vi "TEST_bench_X_minus_Nx_times_ye_singleAxis.vi"(6 "NS + 1":u8=9, 8 "xk_1_2_mem":fxp<+/-,32,5>[](array[numeric])=[0.0, 0.0, 0.0, 0.0, 0.0, 0.0, 0.0, 0.0, 0.0, 0.0, 0.0, 0.0, 0.0, 0.0, 0.0, 0.0, 0.0, 0.0, 0.0, 0.0, 0.0, 0.0, 0.0, 0.0, 0.0, 0.0, 0.0, 0.0, 0.0, 0.0, 0.0, 0.0, 0.0, 0.0, 0.0, 0.0, 0.0, 0.0, 0.0, 0.0, 0.0, 0.0, 0.0, 0.0, 0.0, 0.0, 0.0, 0.0, 0.0, 0.0], 11 "Nx":fxp<+/-,32,5>[](array[numeric])=[0.0, 0.0, 0.0, 0.0, 0.0, 0.0, 0.0, 0.0, 0.0, 0.0, 0.0, 0.0, 0.0, 0.0, 0.0, 0.0, 0.0, 0.0, 0.0, 0.0, 0.0, 0.0, 0.0, 0.0, 0.0, 0.0, 0.0, 0.0, 0.0, 0.0, 0.0, 0.0, 0.0, 0.0, 0.0, 0.0, 0.0, 0.0, 0.0, 0.0, 0.0, 0.0, 0.0, 0.0, 0.0, 0.0, 0.0, 0.0, 0.0, 0.0]) -> ()   [LabVIEW 2017]
uses:
  fpga_subVIs_ssxy/fixed-point-ss/typeDefs/x_control.ctl
  fpga_subVIs_ssxy/fixed-point-ss/typeDefs/Nx_bram.ctl
  fpga_subVIs_ssxy/fixed-point-ss/typeDefs/x_vec_bram.ctl
  <vilib>/rvi/DataTransferAndStorage/Container/Common/niFpgaContainerExecOnDevCompGetState.vi
  <vilib>/rvi/Emulation/niFpgaEmulationIsFPGAContextNoSignature.vi
  <vilib>/rvi/DataTransferAndStorage/Container/Common/niFpgaContainerGetUniqueNameForEmu.vi
  <vilib>/rvi/Emulation/niFpgaProcessEmulError.vi
  <vilib>/rvi/Emulation/niFpgaSctlEmulationGetInTimedLoop.vi
  <vilib>/rvi/errors/nirviReportUnexpectedCaseInternalError (U32).vi
  <vilib>/rvi/Memory/Memory_Emulation/niFpgaMemoryEmulationCacheClearOnFirstRun.vi
  <vilib>/rvi/Memory/Memory_Emulation/nirvimemoryEmulationManagerCache_MakeExclusive.vi
  <vilib>/rvi/Memory/Memory_Emulation/niFpgaMemoryEmulationValidateCache.vi
  <vilib>/rvi/Memory/Memory_Emulation/nirvimemoryEmulationManagerCache_InsertValue.vi
  <vilib>/Utility/error.llb/Clear Errors.vi
  <vilib>/rvi/Memory/Memory_Emulation/nirvimemoryEmulationManagerCache_ReleaseExclusive.vi
  <vilib>/rvi/Memory/Memory_Emulation/nirvimemoryEmulationManagerCache_GetValue.vi
  <vilib>/rvi/Memory/Memory_Emulation/nirvimemoryEmulationManagerCache_SetValue.vi
  <vilib>/rvi/Emulation/niFpgaSctlEmulationResourceMgr.vi
  <vilib>/rvi/DataTransferAndStorage/Container/XNode/niFpgaContainer.xnode
  <vilib>/rvi/Memory/Memory_Emulation/niFpgaMemoryEmulationRefIn.vi
panel:
  out "xerr":T1
  out "x0_expected":fxp<+/-,64,11>[](array[numeric])
  in  "yd_est_x":fxp<+/-,32,5>
  in  "ref(k)_x":fxp<+/-,32,5>
  out "xu_k":fxp<+/-,32,5>
  # "Test that\nxk_1_2 - (r - yd)*Nx"
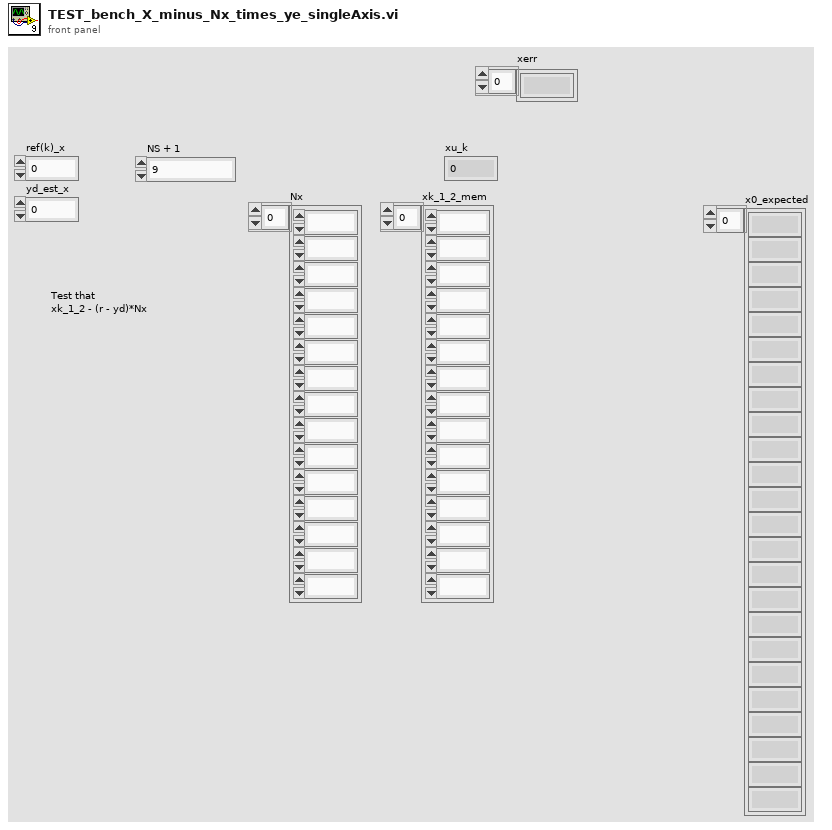
[diagram p1: front panel]
types:
  T1 = typedef "x_control.ctl" = fxp<+/-,18,5>[]
  T2 = typedef "Nx_bram.ctl" = refnum<k21>
  T3 = typedef "x_vec_bram.ctl" = refnum<k21>
  T4 = typedef "x_vec_type.ctl" = fxp<+/-,32,6>[]
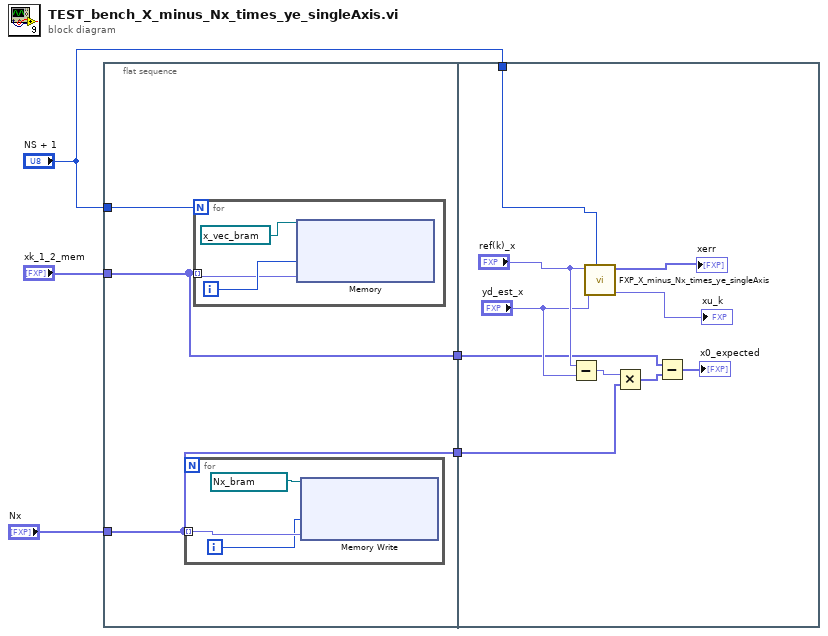
[diagram p0: block diagram]
diagram:
  n1 = flat-sequence {
    tunnel: "NS + 1" -> [w8]
    tunnel: "xk_1_2_mem" -> [w6]
    tunnel: "Nx" -> [w7]
    tunnel: [w7] -> w2
    tunnel: [w6] -> w1
    tunnel: "NS + 1" -> [w24]
    tunnel: w2 -> [w19]
    tunnel: w1 -> [w17]
    frame #0 {
      n2 = for {
        tunnel: w7 -> [w11] mode=indexing
        i -> [w10]
        n3 = xnode "Memory Write"("Address"=w10, "Data"=w11, "Memory In"=T2 "Nx_col1" ("Nx")) -> ()  [unwired: 1 out]
      }
      n4 = for {
        N: w8 -> [_]
        tunnel: w6 -> [w13] mode=indexing
        i -> [w14]
        n5 = xnode "Memory"("Address"=w14, "Data"=w13, "Memory In"=T3 "xk_1_2" ("Memory")) -> ()  [unwired: 1 out]
      }
    }
    frame #1 {
      n6 = Subtract(x="ref(k)_x", y="yd_est_x") -> (x-y=w20:fxp<+/-,33,6>)
      n7 = call "FXP_X_minus_Nx_times_ye_singleAxis.vi"("NS"=w24, "yd_est_x"="yd_est_x", "ref(k)_x"="ref(k)_x") -> ("xu_k"=→"xu_k":fxp<+/-,32,6>, "xerr"=→"xerr":T4)  [unwired: 7 in]
      n8 = Multiply(x=w20, y=w19) -> (x*y=w18:fxp<+/-,64,10>[])
      n9 = Subtract(x=w17, y=w18) -> (x-y=→"x0_expected":fxp<+/-,64,11>[])
    }
  }
